vi "RSZVB Get UI Direction.vi"(8 "error in (no error)":errorcluster {"code" format="%.0x"}, 9 "Port (A)":i32(ring) items=["A", "B", "C", "D"], 11 "VISA session":refnum<visa-resource-name>) -> (0 "error out":errorcluster {"code" format="%.0x"}, 2 "Direction":i32, 3 "dup VISA session":refnum<visa-resource-name>)   [LabVIEW 2011]
doc: "This VI reads the direction of the data flow at ports A, B, C, D. The direction at the combined ports E and F is according to the configuration at the other ports.\n\nRemote-control command(s):\nCONTrol:HANDler:A:MODE?\nCONTrol:HANDler:B:MODE?\nCONTrol:HANDler:C:MODE?\nCONTrol:HANDler:D:MODE?"
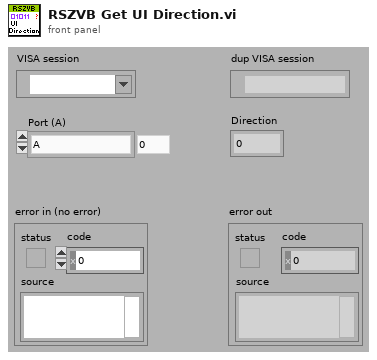
[diagram p1: front panel]
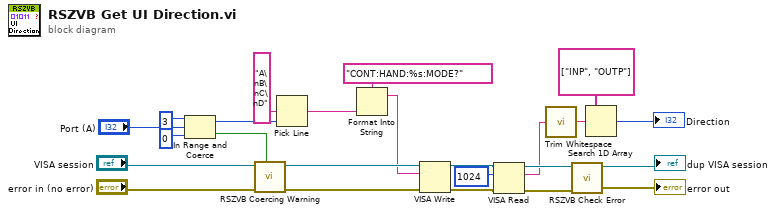
[diagram p0: block diagram]
diagram:
  n1 = In Range and Coerce(upper limit=3, x="Port (A)", lower limit=0) -> (coerced(x)=w17:i32, In Range?=w12:bool)
  n2 = call "RSZVB Coercing Warning.vi"("In Range?"=w12, "error in (no error)"="error in (no error)", "VISA session"="VISA session") -> ("error out"=w22:errorcluster, "dup VISA session"=w23:refnum<visa-resource-name>)  [unwired: 7 in]
  n3 = Pick Line(multi-line string="A\nB\nC\nD", line index=w17) -> (output string=w16:string)  [unwired: 1 in]
  n4 = Format Into String(format string="CONT:HAND:%s:MODE?", w16) -> (resulting string=w21:string)  [unwired: 2 in, 1 out]
  n5 = VISA Write(VISA resource name=w23, write buffer=w21, error in (no error)=w22) -> (VISA resource name out=w5:refnum<visa-resource-name>, error out=w4:errorcluster)  [unwired: 1 out]
  n6 = VISA Read(VISA resource name=w5, byte count=u32 1024 ("byte count (0)"), error in (no error)=w4) -> (VISA resource name out=w10:refnum<visa-resource-name>, read buffer=w6:string, error out=w9:errorcluster)  [unwired: 1 out]
  n7 = call <vilib>:"Trim Whitespace.vi"("string"=w6) -> ("trimmed string"=w7:string)  [unwired: 1 in]
  n8 = call "RSZVB Check Error.vi"("error in (no error)"=w9, "VISA session"=w10) -> ("error out"=→"error out":errorcluster, "dup VISA session"=→"dup VISA session":refnum<visa-resource-name>)  [unwired: 8 in]
  n9 = Search 1D Array(1D array=string[] ["INP", "OUTP"] ("array 2"), element=w7) -> (index of element=→"Direction":i32)  [unwired: 1 in]
